vi "Utility Get Filter Constant.vi"(8 "error in (no error)":errorcluster, 10 "Unit Address (-1)":i32=-1, 11 "VISA resource name (in)":refnum<visa-resource-name>) -> (0 "error out":errorcluster, 2 "Temperature":string, 3 "VISA resource name (out)":refnum<visa-resource-name>)   [LabVIEW 2020]
doc: "Get the current filter constant setting."
uses:
  Omega Platinum Series.lvlib
panel:
  out "Command":string
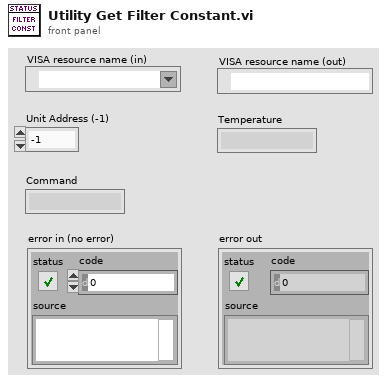
[diagram p1: front panel]
types:
  T1 = typedef "Omega Platinum Series.lvlib/Response.ctl" = cluster{"Unit Address":i32, "Command Class":string, "Command ID":u32, "Parameters":string}
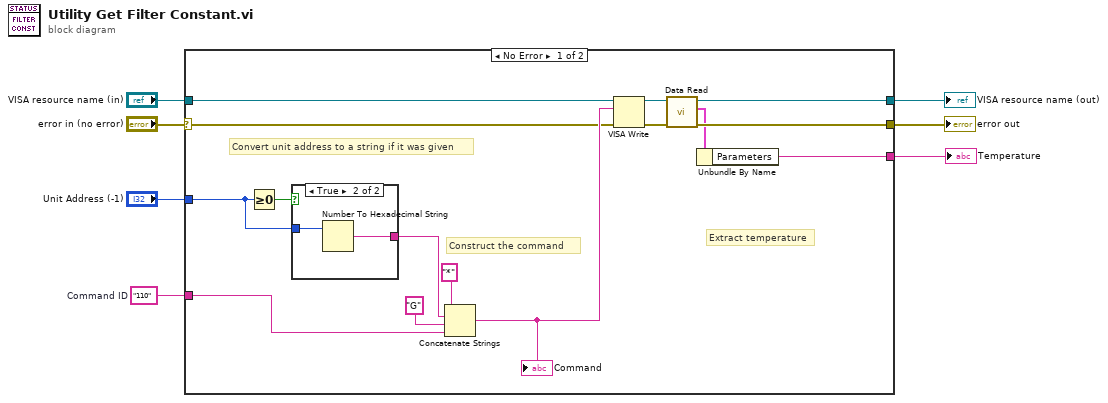
[diagram p0: block diagram]
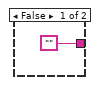
[diagram p2: hidden frame]
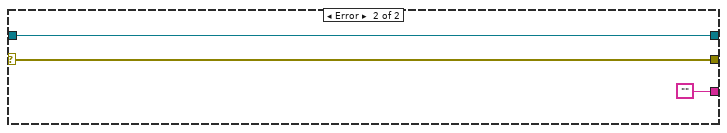
[diagram p3: hidden frame]
diagram:
  w7 = "110"  # Command ID
  n1 = case shown="No Error" "error in (no error)" {
    selector: "error in (no error)" -> [w16 w28]
    tunnel: w7 -> [w10 _]
    tunnel: "Unit Address (-1)" -> [w20 _]
    tunnel: [w12 w28] -> w4
    tunnel: "VISA resource name (in)" -> [w18 w27]
    tunnel: [w13 w27] -> w2
    tunnel: [w8 ""] -> w1
    frame No Error {
      # "Extract temperature"
      # "Convert unit address to a string if it was given"
      # "Construct the command"
      n2 = Greater Or Equal To 0?(x=w20) -> (x >= 0?=w22:bool)
      n3 = case shown="True" w22 {
        tunnel: w20 -> [_ w25]
        tunnel: ["" w24] -> w19
        frame False {
        }
        frame True {
          n4 = Number To Hexadecimal String(2:w25) -> (0:w24:string)  [unwired: 1 in]
        }
      }
      n5 = Concatenate Strings("*" ("string"), w19, "G" ("string"), w10) -> (w17:string)
      "Command" <- w17
      n6 = VISA Write(VISA resource name=w18, write buffer=w17, error in (no error)=w16) -> (VISA resource name out=w14:refnum<visa-resource-name>, error out=w15:errorcluster)  [unwired: 1 out]
      n7 = call "Data Read.vi"("error in (no error)"=w15, "VISA Refnum in"=w14) -> ("error out"=w12:errorcluster, "Response Cluster"=w9:T1, "VISA Refnum out"=w13:refnum<visa-resource-name>)  [unwired: 6 in, 1 out]
      n8 = Unbundle By Name(w9) -> ("Parameters"=w8:string)
    }
    frame Error {
    }
  }
  "error out" <- w4
  "VISA resource name (out)" <- w2
  "Temperature" <- w1
